vi "sub vi - AI USB4704 (3)  Create Task v4.vi"(9 "Rate Hz":dbl, 11 "Samples":dbl) -> (4 "TASK USB 0":i32, 6 "TASK USB 1":i32, 8 "TASK USB 2":i32, 14 "AI Task Er":bool, 15 "error array":errorcluster[](array[cluster]))   [LabVIEW 2017]
uses:
  <userlib>/DAQNavi Polymorphic VI/create/DAQNavi Create Channel(AI-Voltage).vi
  <userlib>/DAQNavi Polymorphic VI/configure/timing/DAQNavi Timing(Convert Clock).vi
  <userlib>/DAQNavi Polymorphic VI/configure/DAQNavi Get Property/AI/DAQNaviGet_AI_ConvertClock_Rate.vi
panel:
  in  "Tab Control":enum32{"Tasks In", "USB #0", "USB #1", "USB #2"}(tab)
  out "physical channels 0":string="DemoDevice,BID#0/ai0:1" caption="property value"
  out "value range 0":string="+/- 5 V" caption="property value"
  out "convert rate 0":dbl
  out "physical channels 1":string="DemoDevice,BID#0/ai0:1" caption="property value"
  out "value range  1":string="+/- 5 V" caption="property value"
  out "convert rate 1":dbl
  out "physical channels 2":string="DemoDevice,BID#0/ai0:1" caption="property value"
  out "value range  2":string="+/- 5 V" caption="property value"
  out "convert rate 2":dbl
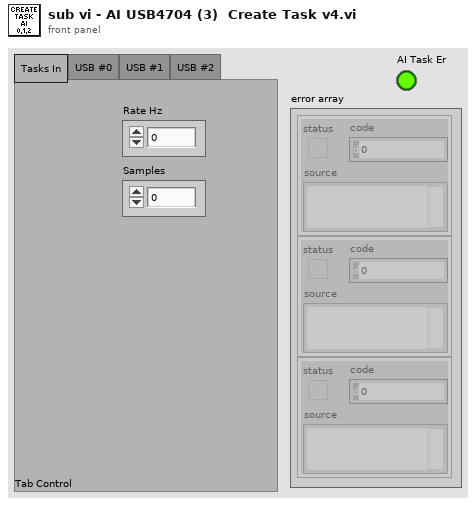
[diagram p1: front panel]
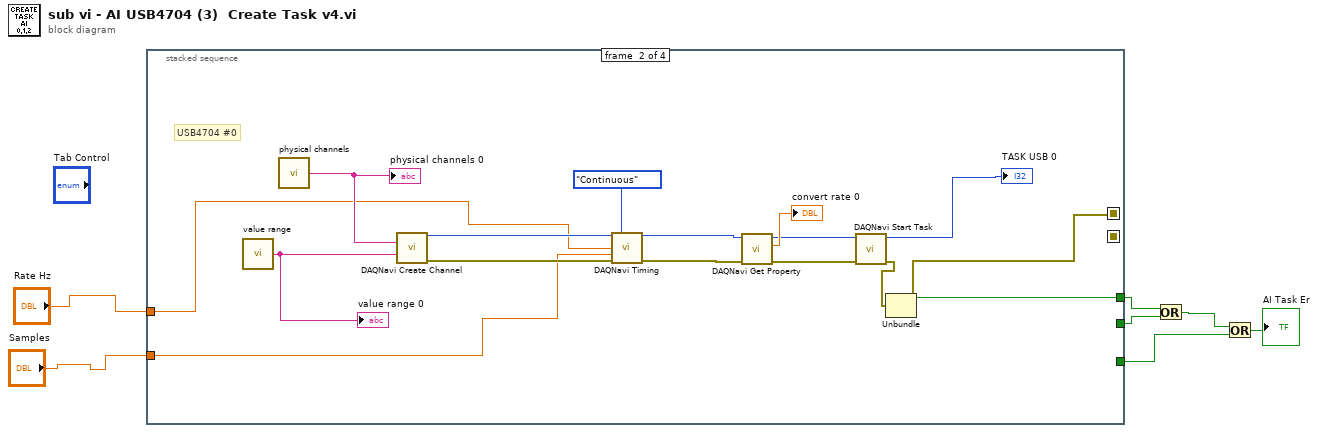
[diagram p0: block diagram]
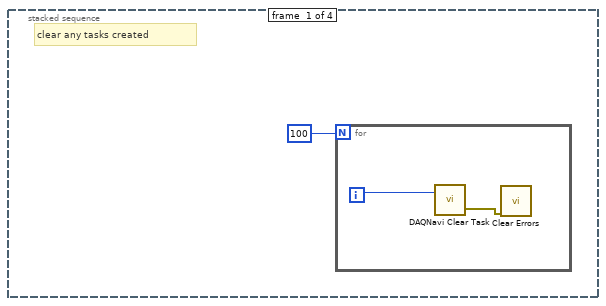
[diagram p2: hidden frame]
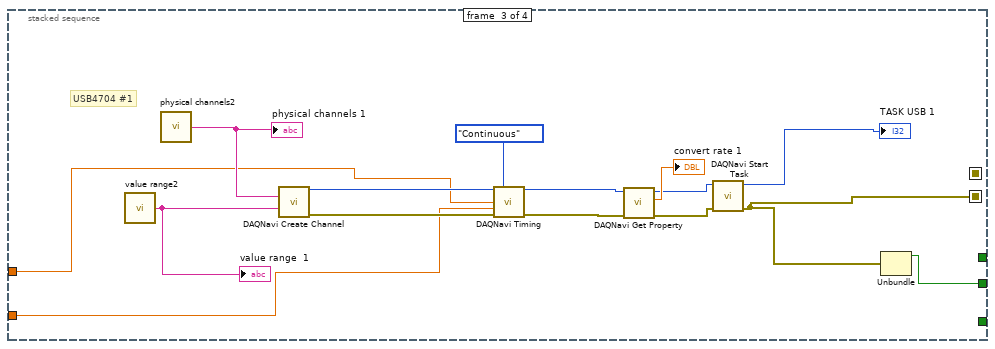
[diagram p3: hidden frame]
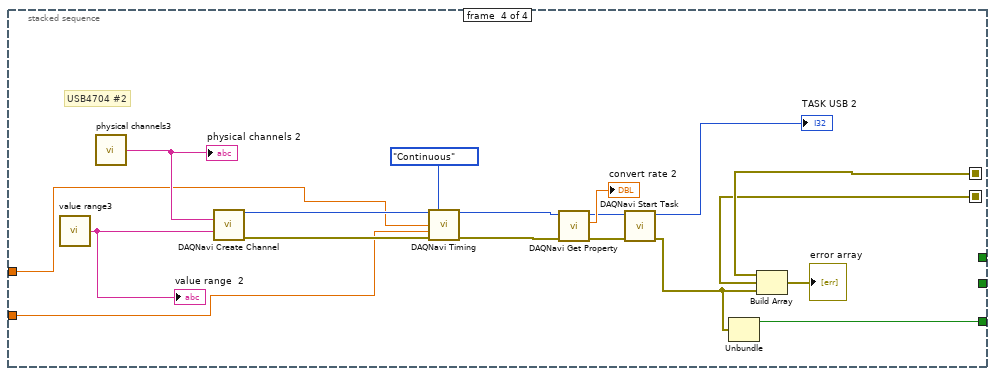
[diagram p4: hidden frame]
diagram:
  n1 = stacked-sequence {
    seq-local: [_ w11 _ _] -> [_ _ _ w50]
    seq-local: [_ _ w27 _] -> [_ _ _ w49]
    tunnel: "Rate Hz" -> [_ w17 w32 w47]
    tunnel: "Samples" -> [_ w16 w31 w46]
    tunnel: [_ _ _ w45] -> w5
    tunnel: [_ w15 _ _] -> w4
    tunnel: [_ _ w30 _] -> w3
    frame #0 {
      # "clear any tasks created"
      n2 = for {
        N: 100 -> [_]
        i -> [w10]
        n3 = call <userlib>:"DAQNavi Clear Task.vi"("task in"=w10) -> ("error out"=w9:errorcluster)  [unwired: 2 in]
        n4 = call <vilib>:"Clear Errors.vi"("error in (no error)"=w9) -> ()  [unwired: 5 in, 2 out]
      }
    }
    frame #1 {
      # "USB4704 #0"
      n5 = call "value range"() -> ("property value"=w25:string)  [unwired: 1 out]
      "value range 0" <- w25
      n6 = call "physical channels"() -> ("property value"=w24:string)  [unwired: 1 out]
      "physical channels 0" <- w24
      n7 = call-poly <userlib>:"DAQNavi Create Channel.vi"("physical channels"=w24, "value range"=w25) -> ("task out"=w18:i32, "error out"=w19:errorcluster)  [unwired: 3 in, 9 out]
      n8 = call-poly <userlib>:"DAQNavi Timing.vi"("task in"=w18, "sample mode"=enum16{"Finite", "Continuous"}."Continuous", "rate"=w17, "samples per channel"=w16, "error in (no error)"=w19) -> ("task out"=w21:i32, "error out"=w22:errorcluster)  [unwired: 1 in, 8 out]
      n9 = call-poly <userlib>:"DAQNavi Get Property.vi"("error in (no error)"=w22, "task in"=w21) -> ("error out"=w14:errorcluster, "rate"=→"convert rate 0":dbl, "task out"=w13:i32)  [unwired: 7 out]
      n10 = call <userlib>:"DAQNavi Start Task.vi"("error in (no error)"=w14, "task in"=w13) -> ("error out"=w11:errorcluster, "task out"=→"TASK USB 0":i32)  [unwired: 8 in]
      n11 = Unbundle(w11) -> ("status"=w15:bool)  [unwired: 2 out]
    }
    frame #2 {
      # "USB4704 #1"
      n12 = call "value range2"() -> ("property value"=w40:string)  [unwired: 1 out]
      "value range  1" <- w40
      n13 = call "physical channels2"() -> ("property value"=w39:string)  [unwired: 1 out]
      "physical channels 1" <- w39
      n14 = call-poly <userlib>:"DAQNavi Create Channel.vi"("physical channels"=w39, "value range"=w40) -> ("task out"=w33:i32, "error out"=w34:errorcluster)  [unwired: 3 in, 9 out]
      n15 = call-poly <userlib>:"DAQNavi Timing.vi"("task in"=w33, "sample mode"=enum16{"Finite", "Continuous"}."Continuous", "rate"=w32, "samples per channel"=w31, "error in (no error)"=w34) -> ("task out"=w36:i32, "error out"=w37:errorcluster)  [unwired: 1 in, 8 out]
      n16 = call-poly <userlib>:"DAQNavi Get Property.vi"("error in (no error)"=w37, "task in"=w36) -> ("error out"=w29:errorcluster, "rate"=→"convert rate 1":dbl, "task out"=w28:i32)  [unwired: 7 out]
      n17 = call <userlib>:"DAQNavi Start Task.vi"("error in (no error)"=w29, "task in"=w28) -> ("error out"=w27:errorcluster, "task out"=→"TASK USB 1":i32)  [unwired: 8 in]
      n18 = Unbundle(w27) -> ("status"=w30:bool)  [unwired: 2 out]
    }
    frame #3 {
      # "USB4704 #2"
      n19 = call "value range3"() -> ("property value"=w58:string)  [unwired: 1 out]
      "value range  2" <- w58
      n20 = call "physical channels3"() -> ("property value"=w57:string)  [unwired: 1 out]
      "physical channels 2" <- w57
      n21 = call-poly <userlib>:"DAQNavi Create Channel.vi"("physical channels"=w57, "value range"=w58) -> ("task out"=w51:i32, "error out"=w52:errorcluster)  [unwired: 3 in, 9 out]
      n22 = call-poly <userlib>:"DAQNavi Timing.vi"("task in"=w51, "sample mode"=enum16{"Finite", "Continuous"}."Continuous", "rate"=w47, "samples per channel"=w46, "error in (no error)"=w52) -> ("task out"=w54:i32, "error out"=w55:errorcluster)  [unwired: 1 in, 8 out]
      n23 = call-poly <userlib>:"DAQNavi Get Property.vi"("error in (no error)"=w55, "task in"=w54) -> ("error out"=w43:errorcluster, "rate"=→"convert rate 2":dbl, "task out"=w44:i32)  [unwired: 7 out]
      n24 = call <userlib>:"DAQNavi Start Task.vi"("error in (no error)"=w43, "task in"=w44) -> ("error out"=w42:errorcluster, "task out"=→"TASK USB 2":i32)  [unwired: 8 in]
      n25 = Unbundle(w42) -> ("status"=w45:bool)  [unwired: 2 out]
      n26 = Build Array(w50, w49, w42) -> (→"error array":errorcluster[])
    }
  }
  n27 = Or(x=w4, y=w3) -> (x .or. y?=w6:bool)
  n28 = Or(x=w6, y=w5) -> (x .or. y?=→"AI Task Er":bool)
